vi "Create_API_Reference.vi"(2 "API Function Array In":cluster{string, "VI Reference":refnum<vi>}[](array[cluster]), 3 "ID":string, 4 "Command":string) -> (0 "API Function Array Out":cluster{string, "VI Reference":refnum<vi>}[](array[cluster]), 1 "VI Reference":refnum<vi>)   [LabVIEW 2011]
doc: "This VI creates a new API VI reference based on the polymorphic API VI specification that can be seen in the Example.vi file in the \"api\" directory. This is needed for every API event start/end pair in the sequence."
panel:
  out "Error Out":errorcluster
  in  "Type Specifier":refnum<vi>
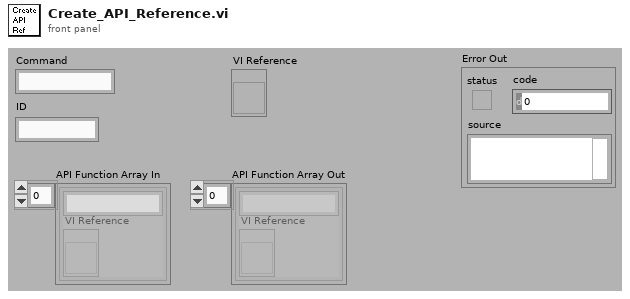
[diagram p1: front panel]
types:
  T1 = cluster{"ID":string, "Type Specifier":refnum<vi>}
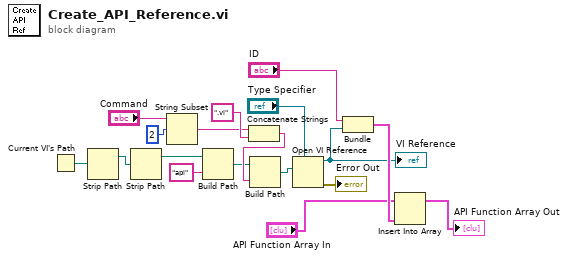
[diagram p0: block diagram]
diagram:
  n1 = Current VI's Path() -> (path=w3:path)
  n2 = Strip Path(path=w3) -> (stripped path=w2:path)  [unwired: 1 out]
  n3 = Strip Path(path=w2) -> (stripped path=w10:path)  [unwired: 1 out]
  n4 = String Subset(string="Command", offset (0)=2) -> (substring=w14:string)  [unwired: 1 out]
  n5 = Build Path(base path=w10, name or relative path="api") -> (appended path=w16:path)
  n6 = Concatenate Strings(w14, ".vi" ("string")) -> (w17:string)
  n7 = Build Path(base path=w16, name or relative path=w17) -> (appended path=w12:path)
  n8 = Open VI Reference(type specifier VI Refnum (for type only)="Type Specifier", vi path=w12) -> (vi reference=w7:refnum<vi>, error out=→"Error Out":errorcluster)  [unwired: 2 in, 2 out]
  "VI Reference" <- w7
  n9 = Bundle("ID"="ID", "Type Specifier"=w7) -> (w11:T1)  [unwired: 1 out]
  n10 = Insert Into Array(array="API Function Array In", new element=w11) -> (→"API Function Array Out":cluster{string, "VI Reference":refnum<vi>}[])  [unwired: 1 in]
